vi "Result_Test.vi"(8 "error in (no error)":errorcluster caption="entrée d'erreur (pas d'erreur)", 11 "Generate_SN en entrée":refnum<class "Nodon_Generate_SN_Product.lvclass">) -> (0 "error out":errorcluster caption="sortie d'erreur", 3 "Generate_SN en sortie":refnum<class "Nodon_Generate_SN_Product.lvclass">)   [LabVIEW 2020, in "Library Test.lvlib" / "Nodon_Generate_SN_Product.lvclass"]
uses:
  Nodon_Generate_SN_Product.lvclass
  C:/Users/ngarcin/OneDrive - Altyor/Standard TB/Suite TB45/Class/Test/Find_SN_In_Database/Find_SN_In_Database.lvclass
  Commun VI/TypeDef/Variable Printable.ctl
  Find_SN_In_Database/Find_SN_In_Database.lvclass
  Commun VI/Library Commun.lvlib
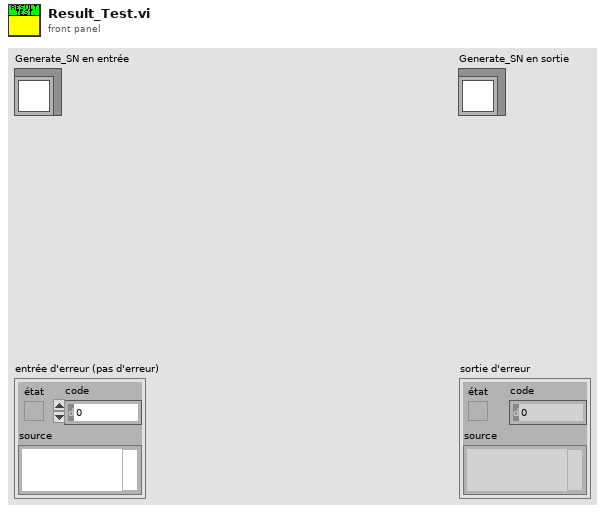
[diagram p1: front panel]
types:
  T1 = typedef "Variable Printable.ctl" = string
  T2 = enum16{"Get Variable", "Get All Variables", "Set Variable", "Delete Variable", "Delete All Variable"}
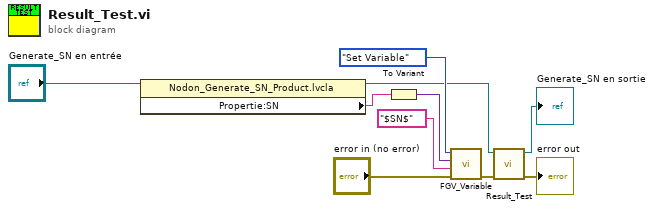
[diagram p0: block diagram]
diagram:
  n1 = property class="Nodon_Generate_SN_Product.lvcla"(reference="Generate_SN en entrée") -> (reference out=w2:refnum<class "Nodon_Generate_SN_Product.lvclass">, "Propertie:SN"=w5:string)  [unwired: 1 in, 1 out]
  n2 = To Variant(anything=w5) -> (Variant=w7:variant)
  n3 = call "FGV_Variable.vi"("error in (no error)"="error in (no error)", "Variable"=T1 "$SN$", "Data In"=w7, "Function"=T2."Set Variable") -> ("error out"=w1:errorcluster)  [unwired: 5 in, 2 out]
  n4 = call-parent "Result_Test.vi"("error in (no error)"=w1, "Generate_SN en entrée"=w2) -> ("error out"=→"error out":errorcluster, "Generate_SN en sortie"=→"Generate_SN en sortie":refnum<class "Nodon_Generate_SN_Product.lvclass">)  [unwired: 8 in]
